vi "set_gate_parameters.vi"(4 "repetitions":i64, 5 "pulse duration (iterations)":i64, 6 "offset duration (iterations)":i64, 7 "clock index":i32, 8 "error in (no error)":errorcluster, 9 "low phase duration (iterations)":i64, 10 "high phase duration (iterations)":i64, 11 "FPGAWrapperDL090211Galvo in":refnum<class "FPGAWrapperDL090211Galvo.lvclass">) -> (0 "error out":errorcluster, 3 "FPGAWrapperDL090211Galvo out":refnum<class "FPGAWrapperDL090211Galvo.lvclass">)   [LabVIEW 2010, in "FPGAWrapperDL090211Galvo.lvclass"]
uses:
  FPGAWrapperDL090211Galvo.lvclass
  common_typedefs/gate_parameters_cluster.ctl
  <vilib>/rvi/interface/nirviReadWriteControl/nirviReadWriteControl.xnode
  FPGA_VI_ref.ctl
  <vilib>/rvi/interface/common/niFpgaNodeNameForErrorReporting.ctl
  <vilib>/rvi/errors/niLvFpgaWhatHappensToTopLevelVI.ctl
  <vilib>/Utility/error.llb/Error Cluster From Error Code.vi
  <vilib>/rvi/errors/niLvFpgaAdjustHostInterfaceError.vi
  NiFpgaLv.dll
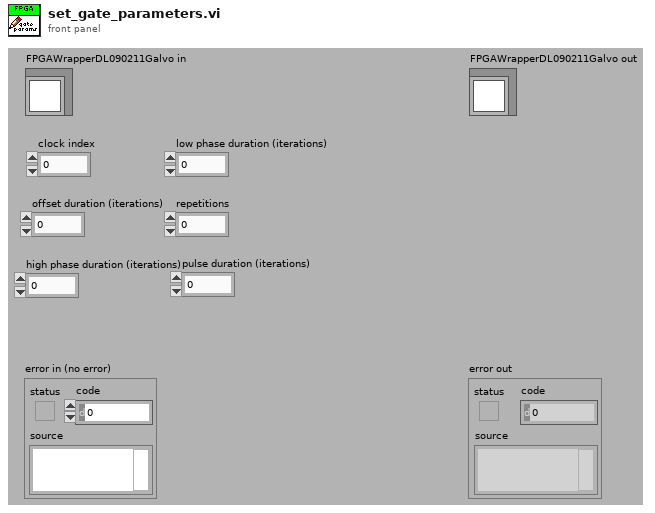
[diagram p1: front panel]
types:
  T1 = typedef "gate_parameters_cluster.ctl" = cluster{"offset":i64, "pulsing":i64, "not pulsing":i64, "cycles per pulse":i64, "repetitions":i64}
  T2 = typedef "niFpgaNodeNameForErrorReporting.ctl" = enum16{"Open FPGA VI Reference", "Read/Write Control", "Invoke Method: Abort", "Invoke Method: Acknowledge IRQ", "Invoke Method: Download", "Invoke Method: FIFO.Configure", "Invoke Method: FIFO.Read", "Invoke Method: FIFO.Start", "Invoke Method: FIFO.Stop", "Invoke Method: FIFO.Write", "Invoke Method: Reset", "Invoke Method: Run", "Invoke Method: Wait on IRQ", "Close FPGA VI Reference"}
  T3 = typedef "niLvFpgaWhatHappensToTopLevelVI.ctl" = enum16{"top level VI scripted behind XNode", "top level VI inlined behind XNode"}
  T4 = typedef "FPGAWrapperDL090211Galvo.lvclass/FPGA_VI_ref.ctl" = refnum<k20>
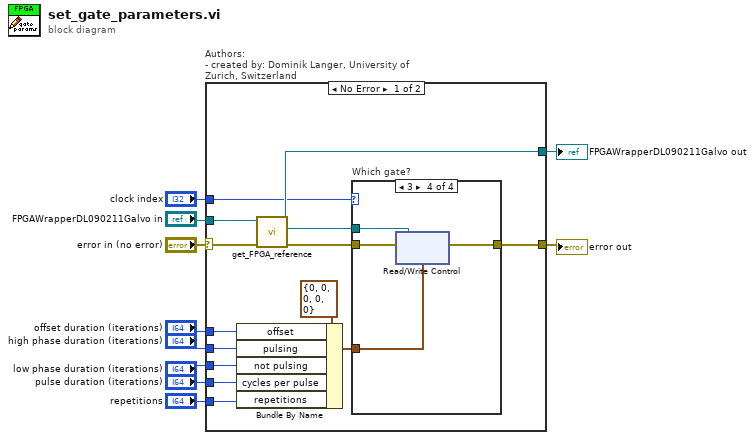
[diagram p0: block diagram]
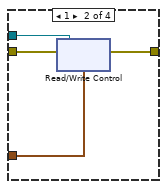
[diagram p3: hidden frame]
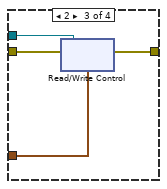
[diagram p4: hidden frame]
diagram:
  n1 = case "Authors: \n- created by: Dominik Langer, University of Zurich, Switzerland" shown="No Error" "error in (no error)" {
    selector: "error in (no error)" -> [w19 w170]
    tunnel: "FPGAWrapperDL090211Galvo in" -> [w24 w171]
    tunnel: [w23 w171] -> w9
    tunnel: [w20 w170] -> w8
    tunnel: "clock index" -> [w18 _]
    tunnel: "repetitions" -> [w15 _]
    tunnel: "high phase duration (iterations)" -> [w14 _]
    tunnel: "offset duration (iterations)" -> [w13 _]
    tunnel: "low phase duration (iterations)" -> [w12 _]
    tunnel: "pulse duration (iterations)" -> [w11 _]
    frame No Error {
      n2 = Bundle By Name(cluster=T1 {"offset"=0, "pulsing"=0, "not pulsing"=0, "cycles per pulse"=0, "repetitions"=0} ("gate 1"), "offset"=w13, "pulsing"=w14, "not pulsing"=w12, "cycles per pulse"=w11, "repetitions"=w15) -> (w16:T1)
      n3 = call-dynamic "get_FPGA_reference.vi"("error in (no error)"=w19, "FPGAWrapperDL090211Galvo in"=w24) -> ("error out"=w22:errorcluster, "FPGA VI reference"=w21:T4, "FPGAWrapperDL090211Galvo out"=w23:refnum<class "FPGAWrapperDL090211Galvo.lvclass">)  [unwired: 6 in, 1 out]
      n4 = case "Which gate?" shown="3" w18 {
        tunnel: w22 -> [w25 w29 w76 w123]
        tunnel: w21 -> [_ w28 w77 w125]
        tunnel: [w25 w27 w75 w122] -> w20
        tunnel: w16 -> [_ w26 w74 w124]
        frame Default {
        }
        frame 1 {
          n5 = xnode "Read/Write Control"("FPGA VI Reference In"=w28, "error in"=w29, "gate 1"=w26) -> ("error out"=w27:errorcluster)  [unwired: 1 out]
        }
        frame 2 {
          n6 = xnode "Read/Write Control"("FPGA VI Reference In"=w77, "error in"=w76, "gate 2"=w74) -> ("error out"=w75:errorcluster)  [unwired: 1 out]
        }
        frame 3 {
          n7 = xnode "Read/Write Control"("FPGA VI Reference In"=w125, "error in"=w123, "gate 3"=w124) -> ("error out"=w122:errorcluster)  [unwired: 1 out]
        }
      }
    }
    frame Error {
    }
  }
  "error out" <- w8
  "FPGAWrapperDL090211Galvo out" <- w9
